vi "VISA BAR3 Read U8 vs U64.vi"() -> ()   [LabVIEW 2016]
uses:
  <vilib>/Platform/TimedLoop/XDataNode/timing_clust.ctl
  <vilib>/Platform/TimedLoop/XDataNode/nitl_modes.ctl
  <vilib>/Platform/TimedLoop/XDataNode/wakeup.ctl
  Source/GE 5565PIORC/GE 5565PIORC.lvclass/GE 5565PIORC.ctl
  <vilib>/Instr/_visa.llb/VISA Register Access Address Space.ctl
  Source/GE 5565PIORC/VIs/Registers/Local Configuration.LAS1RR.Address Range.Get.vi
  Source/GE 5565PIORC/VIs/Registers/Local Configuration.Get Register Offset.vi
  Source/GE 5565PIORC/GE 5565PIORC.lvclass
  <vilib>/platform/TimedLoop/XDataNode/XDataNode.xnode
  <vilib>/Platform/TimedLoop/XDataNode/XDNodeRunTimeDep.lvlib
panel:
  out "U64 Duration":dbl
  in  "U64s":i32
  out "U8 Duration":dbl
  in  "VISA resource name":refnum<visa-resource-name>
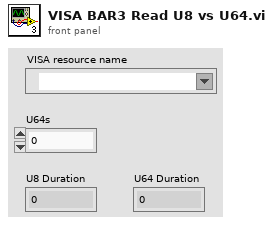
[diagram p1: front panel]
types:
  T1 = typedef "XDNodeRunTimeDep.lvlib/timing_clust.ctl" = cluster{"Expected End [f-1]":u64, "Actual End [f-1]":u64, "Finished Late? [f-1]":bool, "Expected End [i-1]":u64, "Actual End [i-1]":u64, "Finished Late? [i-1]":bool, "Expected Start [i]":u64, "Actual Start [i]":u64, "Expected Start [f]":u64, "Actual Start [f]":u64, "Source Name":string, "Structure Name":string, "Period":i64, "Deadline":i64, "Offset":i64, "Start":i64, "Priority":i32, "Timeout":i32, "Mode":T2, "Wakeup Reason":T3, "Error":errorcluster, "Source Type":string, "Secondary Source Type":string, "Global End Time":u64, "Global Start Time":u64, "Frame Duration":u64, "Iteration Duration":u64, "Assigned CPU":i32, "I/O Scan Engine Mode":u32}
  T2 = typedef "XDNodeRunTimeDep.lvlib/nitl_modes.ctl" = enum32{"No Change", "Process missed periods, maintain original phase", "Discard missed periods, maintain original phase", "Process missed periods, ignore original phase", "Discard missed periods, ignore original phase"}
  T3 = typedef "XDNodeRunTimeDep.lvlib/wakeup.ctl" = enum32{"Normal", "Aborted", "Asynchronous wakeup", "Timing source error", "Timed loop error", "Timeout"}
  T4 = typedef "VISA Register Access Address Space.ctl" = u16
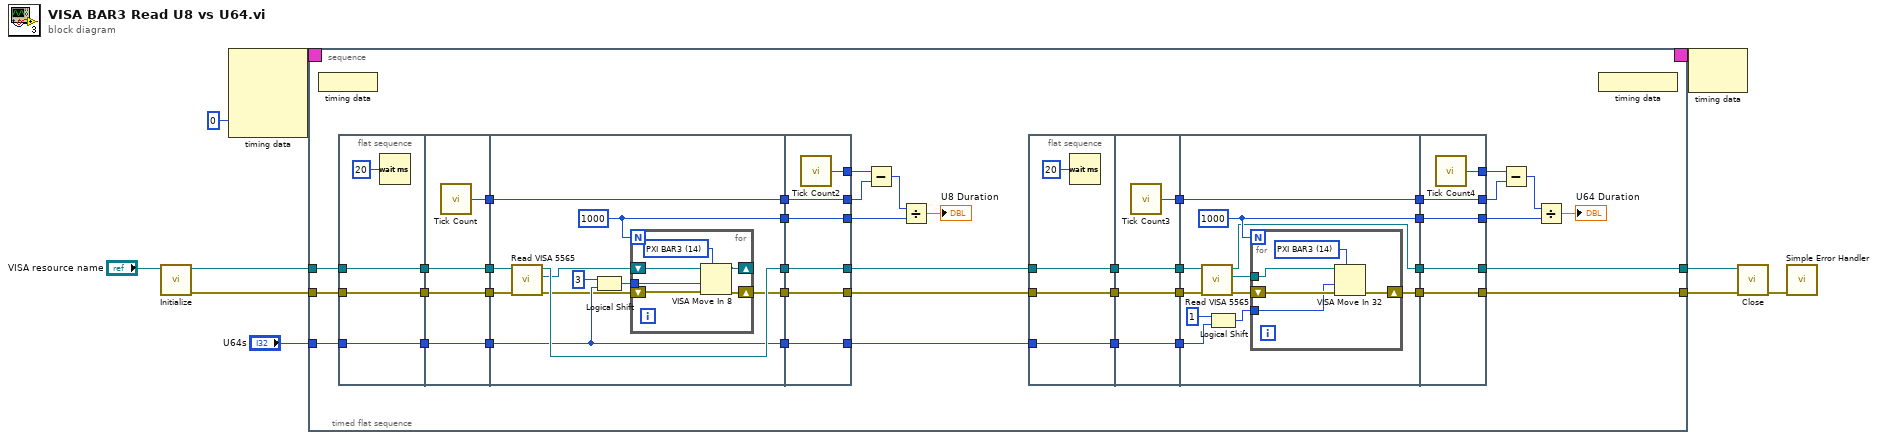
[diagram p0: block diagram]
diagram:
  n1 = call "Initialize.vi"("VISA resource name"="VISA resource name") -> ("error out"=w4:errorcluster, "GE 5565PIORC"=w5:refnum<class "GE 5565PIORC.lvclass">)  [unwired: 9 in]
  n2 = node-c288(0 ("Processor")) -> (w8:T1)  [unwired: 3 in]
  n3 = timed-sequence {
    timing: w8 -> [_]
    timing-out: [_] -> w7
    tunnel: w5 -> [w15]
    tunnel: w4 -> [w14]
    tunnel: [w12] -> w3
    tunnel: [w11] -> w2
    tunnel: "U64s" -> [w13]
    n4 = timed-flat-sequence {
      tunnel: w15 -> [w52]
      tunnel: w14 -> [w51]
      tunnel: w13 -> [w40]
      tunnel: [w20] -> w12
      tunnel: [w19] -> w11
      n5 = node-c288() -> ()  [unwired: 1 in]
      n6 = flat-sequence {
        tunnel: w52 -> [w88]
        tunnel: w51 -> [w87]
        tunnel: [w88] -> w49
        tunnel: [w87] -> w47
        tunnel: w40 -> [w86]
        tunnel: [w86] -> w38
        tunnel: [w93] -> w56
        tunnel: [w92] -> w50
        tunnel: w49 -> [w92]
        tunnel: [w91] -> w48
        tunnel: w47 -> [w91]
        tunnel: [w90] -> w39
        tunnel: w38 -> [w90]
        tunnel: w56 -> [w104]
        tunnel: [w104] -> w55
        tunnel: w50 -> [w103]
        tunnel: w48 -> [w96]
        tunnel: [w102] -> w46
        tunnel: [w101] -> w45
        tunnel: [w100] -> w44
        tunnel: w39 -> [w99]
        tunnel: [w99] -> w18
        tunnel: [w116] -> w54
        tunnel: [w115] -> w53
        tunnel: w55 -> [w115]
        tunnel: w46 -> [w114]
        tunnel: w45 -> [w113]
        tunnel: [w114] -> w22
        tunnel: [w113] -> w21
        tunnel: w44 -> [w112]
        tunnel: [w112] -> w42
        tunnel: w18 -> [w111]
        tunnel: [w111] -> w17
        frame #0 {
          n7 = Wait (ms)(milliseconds to wait=u32 20) -> ()  [unwired: 1 out]
        }
        frame #1 {
          n8 = call "Tick Count"() -> ("Tick Count(uSec)"=w93:u32)
        }
        frame #2 {
          w100 = 1000
          n9 = call "Read VISA 5565.vi"("error in (no error)"=w96, "GE 5565PIORC in"=w103) -> ("error out"=w94:errorcluster, "VISA 5565"=w95:refnum<visa-resource-name>, "GE 5565PIORC out"=w102:refnum<class "GE 5565PIORC.lvclass">)  [unwired: 7 in]
          n10 = Logical Shift(y=i16 3, x=w99) -> (x << y=w98:i32)
          n11 = for {
            N: w100 -> [_]
            shift-right: [w108] -> _
            shift-left: w95 -> [w109]
            shift-right: [w107] -> w101
            shift-left: w94 -> [w106]
            tunnel: w98 -> [w105]
            w110 = T4 14 items=["VXI/VME A16"=1, "VXI/VME A24"=2, "VXI/VME A32"=3, "VXI/VME A64"=4, "PXI Memory Allocations"=9, "PXI Configuration"=10, "PXI BAR0"=11, "PXI BAR1"=12, "PXI BAR2"=13, "PXI BAR3"=14, "PXI BAR4"=15, "PXI BAR5"=16] ("Address Space")
            n12 = VISA Move In 8(7:w110, 8:w106, 9:w105, 11:w109) -> (0:w107:errorcluster, 3:w108:refnum<visa-resource-name>)  [unwired: 1 in, 1 out]
          }
        }
        frame #3 {
          n13 = call "Tick Count2"() -> ("Tick Count(uSec)"=w116:u32)
        }
      }
      n14 = Subtract(x=w54, y=w53) -> (x-y=w43:u32)
      n15 = Divide(x=w43, y=w42) -> (x/y=→"U8 Duration":dbl)
      n16 = flat-sequence {
        tunnel: w22 -> [w59]
        tunnel: w21 -> [w58]
        tunnel: [w59] -> w37
        tunnel: [w58] -> w36
        tunnel: w17 -> [w57]
        tunnel: [w57] -> w35
        tunnel: [w64] -> w34
        tunnel: [w63] -> w33
        tunnel: w37 -> [w63]
        tunnel: [w62] -> w32
        tunnel: w36 -> [w62]
        tunnel: [w61] -> w31
        tunnel: w35 -> [w61]
        tunnel: w34 -> [w75]
        tunnel: [w75] -> w30
        tunnel: w33 -> [w72]
        tunnel: w32 -> [w71]
        tunnel: [w74] -> w29
        tunnel: [w73] -> w28
        tunnel: w31 -> [w66]
        tunnel: [w68] -> w16
        tunnel: [w85] -> w27
        tunnel: [w84] -> w26
        tunnel: w30 -> [w84]
        tunnel: w29 -> [w83]
        tunnel: [w81] -> w20
        tunnel: [w83] -> w19
        tunnel: w28 -> [w82]
        tunnel: [w82] -> w24
        tunnel: w16 -> [w81]
        frame #0 {
          n17 = Wait (ms)(milliseconds to wait=u32 20) -> ()  [unwired: 1 out]
        }
        frame #1 {
          n18 = call "Tick Count3"() -> ("Tick Count(uSec)"=w64:u32)
        }
        frame #2 {
          w73 = 1000
          n19 = call "Read VISA 5565.vi"("error in (no error)"=w71, "GE 5565PIORC in"=w72) -> ("error out"=w70:errorcluster, "VISA 5565"=w69:refnum<visa-resource-name>, "GE 5565PIORC out"=w68:refnum<class "GE 5565PIORC.lvclass">)  [unwired: 7 in]
          n20 = Logical Shift(y=i16 1, x=w66) -> (x << y=w65:i32)
          n21 = for {
            N: w73 -> [_]
            shift-right: [w79] -> w74
            shift-left: w70 -> [w80]
            tunnel: w65 -> [w78]
            tunnel: w69 -> [w76]
            w77 = T4 14 items=["VXI/VME A16"=1, "VXI/VME A24"=2, "VXI/VME A32"=3, "VXI/VME A64"=4, "PXI Memory Allocations"=9, "PXI Configuration"=10, "PXI BAR0"=11, "PXI BAR1"=12, "PXI BAR2"=13, "PXI BAR3"=14, "PXI BAR4"=15, "PXI BAR5"=16] ("Address Space")
            n22 = VISA Move In 32(7:w77, 8:w80, 9:w78, 11:w76) -> (0:w79:errorcluster)  [unwired: 1 in, 2 out]
          }
        }
        frame #3 {
          n23 = call "Tick Count4"() -> ("Tick Count(uSec)"=w85:u32)
        }
      }
      n24 = Subtract(x=w27, y=w26) -> (x-y=w25:u32)
      n25 = Divide(x=w25, y=w24) -> (x/y=→"U64 Duration":dbl)
      n26 = node-c288() -> ()  [unwired: 1 out]
    }
  }
  n27 = node-c288(w7) -> ()  [unwired: 1 out]
  n28 = call "Close.vi"("error in (no error)"=w2, "GE 5565PIORC in"=w3) -> ("error out"=w9:errorcluster)  [unwired: 8 in, 1 out]
  n29 = call <vilib>:"Simple Error Handler.vi"("error in (no error)"=w9) -> ()  [unwired: 4 in, 5 out]
